vi "PhysMon-Append To Data Log.vi"(0 "Timestamp":timestamp, 1 "Path":path, 5 "Heart Rate (bpm)":dbl, 7 "Temperature (C)":dbl, 9 "Note":string, 11 "error in (no error)":errorcluster) -> (15 "error out":errorcluster)   [LabVIEW 2020]
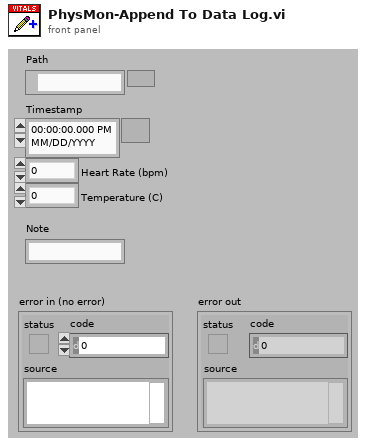
[diagram p1: front panel]
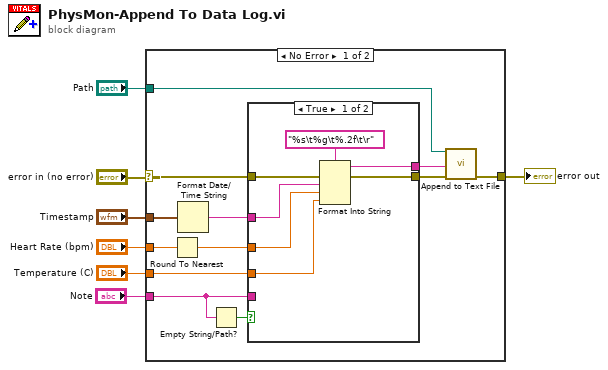
[diagram p0: block diagram]
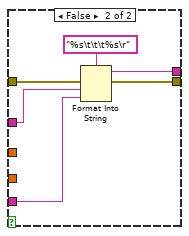
[diagram p2: hidden frame]
diagram:
  n1 = case shown="No Error" "error in (no error)" {
    selector: "error in (no error)" -> [w19 w33]
    tunnel: [w10 w33] -> w6
    tunnel: "Timestamp" -> [w18 _]
    tunnel: "Heart Rate (bpm)" -> [w16 _]
    tunnel: "Temperature (C)" -> [w14 _]
    tunnel: "Path" -> [w11 _]
    tunnel: "Note" -> [w8 _]
    frame No Error {
      n2 = Round To Nearest(number=w16) -> (nearest integer value=w15:dbl)
      n3 = Format Date/Time String(seconds (now)=w18) -> (date/time string=w17:string)  [unwired: 2 in]
      n4 = Empty String/Path?(string/path=w8) -> (empty?=w9:bool)
      n5 = case shown="True" w9 {
        tunnel: w19 -> [w25 w31]
        tunnel: w17 -> [w24 w28]
        tunnel: w15 -> [w23 _]
        tunnel: w14 -> [w22 _]
        tunnel: [w21 w30] -> w13
        tunnel: [w20 w29] -> w12
        tunnel: w8 -> [_ w27]
        frame True {
          n6 = Format Into String(format string="%s\t%g\t%.2f\t\r", error in=w25, w24, w23, w22) -> (resulting string=w20:string, error out=w21:errorcluster)  [unwired: 1 in]
        }
        frame False {
          n7 = Format Into String(format string="%s\t\t\t%s\r", error in=w31, w28, w27) -> (resulting string=w29:string, error out=w30:errorcluster)  [unwired: 1 in]
        }
      }
      n8 = call "Append to Text File.vi"("file path"=w11, "text"=w12, "error in (no error)"=w13) -> ("error out"=w10:errorcluster)  [unwired: 11 in, 1 out]
    }
    frame Error {
    }
  }
  "error out" <- w6
